vi "Create Message_TriggerOnly.vi"(4 "Trigger Channel refnum":T1=18446744073709551615 format="%.0x", 6 "Enable Periodic Default ON":bool, 8 "error in (no error)":errorcluster, 9 "Protection":T2(ring), 10 "Message name":string, 11 "Message Group refnum in":T1=18446744073709551615 format="%.0x") -> (0 "error out":errorcluster, 2 "Message refnum out":T1=18446744073709551615 format="%.0x", 3 "Message Group refnum out":T1=18446744073709551615 format="%.0x")   [LabVIEW 2019, in "Scripting API.lvlib"]
uses:
  Scripting API.lvlib
  <vilib>/NI VeriStand/Custom Device API/Custom Device Item Ref.ctl
  <vilib>/NI VeriStand/Custom Device API/Custom Device API.lvlib
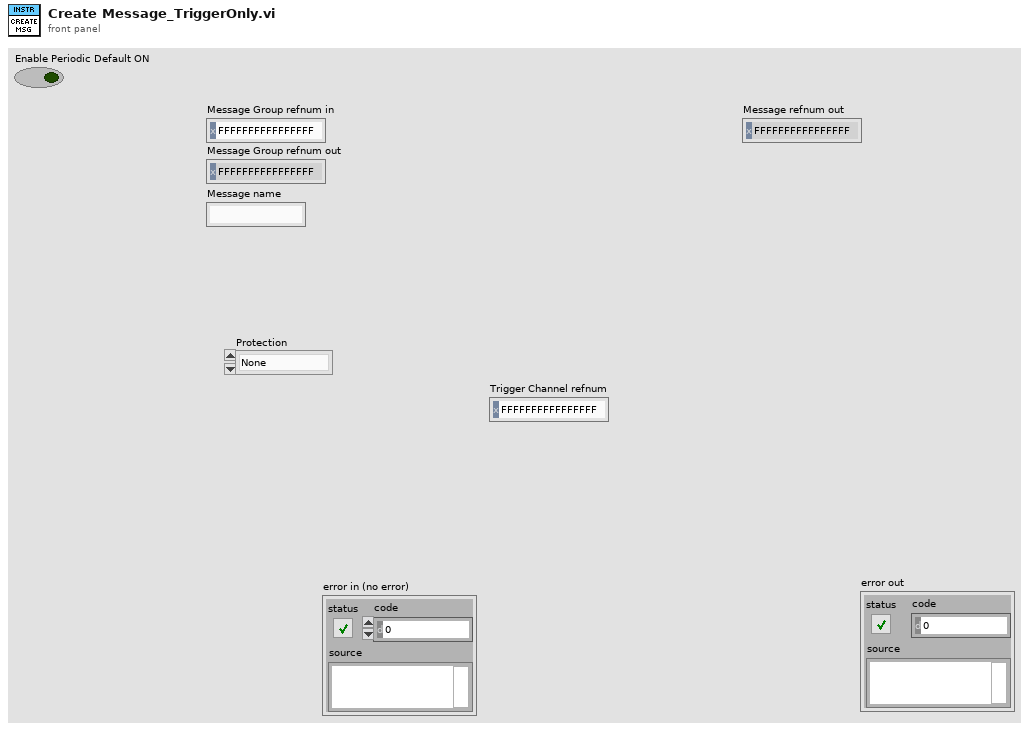
[diagram p1: front panel]
types:
  T1 = typedef "Custom Device API.lvlib/Custom Device Item Ref.ctl" = u64
  T2 = enum16{"None", "CRC-32", "Checksum U8", "Checksum U16", "Checksum U32"}
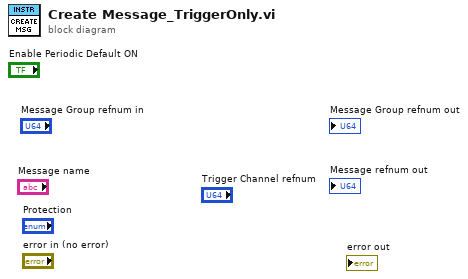
[diagram p0: block diagram]
diagram:
